vi "read_DAC.vi"() -> ()   [LabVIEW 2014]
uses:
  aardvark.dll
panel:
  out "Dup Aardvark Handle":i32
  out "DAC Val":u16 format="%.0x"
  in  "DAC_ADD":u16[](array[numeric]) format="%.0x"
  out "error out":errorcluster
  in  "error in (no error)":errorcluster
  in  "Address (0x50)":u16=80 max=1023 format="%.0x"
  in  "Aardvark Handle":i32 min=0
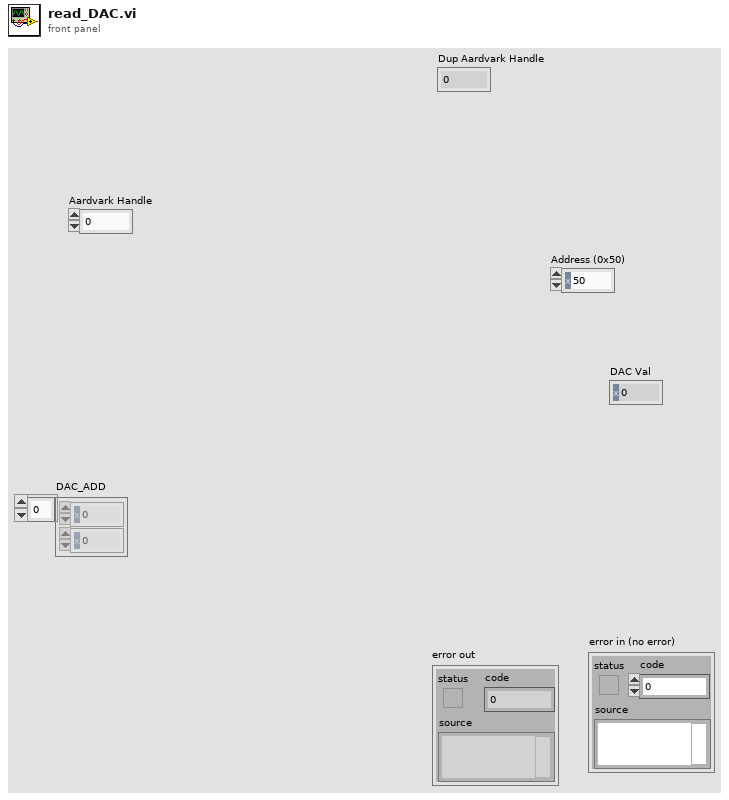
[diagram p1: front panel]
types:
  T1 = cluster{"Boolean array[0]":bool, "Boolean array[1]":bool, "Boolean array[2]":bool, "Boolean array[3]":bool, "Boolean array[4]":bool, "Boolean array[5]":bool, "Boolean array[6]":bool, "Boolean array[7]":bool}
  T2 = cluster{"Boolean array[0]":bool, "Boolean array[1]":bool, "Boolean array[2]":bool, "Boolean array[3]":bool, "Boolean array[4]":bool, "Boolean array[5]":bool, "Boolean array[6]":bool, "Boolean array[7]":bool, "Boolean array[0]":bool, "Boolean array[1]":bool, "Boolean array[2]":bool, "Boolean array[3]":bool}
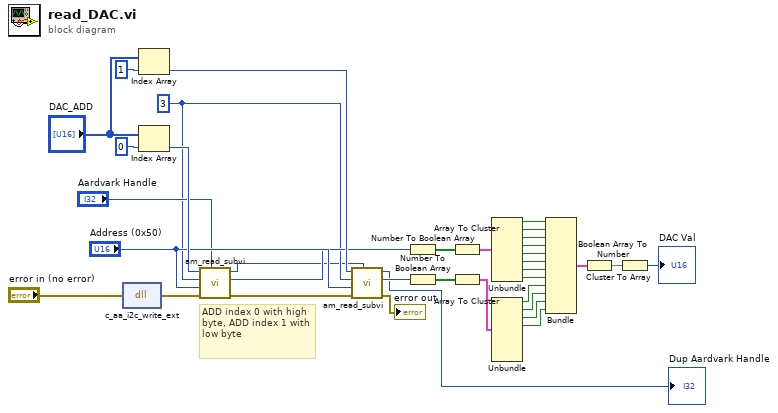
[diagram p0: block diagram]
diagram:
  w3 = u8 3
  # "ADD index 0 with high byte, ADD index 1 with low byte"
  n1 = dll-call lib="aardvark.dll" fn="c_aa_i2c_write_ext"(error in="error in (no error)") -> (error out=w30:errorcluster)  [unwired: 3 in, 1 out]
  n2 = Index Array(array="DAC_ADD", index=1) -> (element=w26:u16)
  n3 = Index Array(array="DAC_ADD", index=0) -> (element=w31:u16)
  n4 = call "am_read_subvi.vi"("Aardvark Handle in"="Aardvark Handle", "error in (no error)"=w30, "Address (0x50) in"="Address (0x50)", "Num Bytes to Fetch (64)"=w3, "Memory ADD"=w31) -> ("error out"=w29:errorcluster, "Data byte"=w4:u8, "Dup Aardvark Handle"=w2:i32)  [unwired: 4 in]
  n5 = call "am_read_subvi.vi"("Aardvark Handle in"=w2, "error in (no error)"=w29, "Address (0x50) in"="Address (0x50)", "Num Bytes to Fetch (64)"=w3, "Memory ADD"=w26) -> ("error out"=→"error out":errorcluster, "Data byte"=w5:u8, "Dup Aardvark Handle"=→"Dup Aardvark Handle":i32)  [unwired: 4 in]
  n6 = Number To Boolean Array(number=w4) -> (Boolean array=w23:bool[])
  n7 = Number To Boolean Array(number=w5) -> (Boolean array=w21:bool[])
  n8 = Array To Cluster(array=w23) -> (cluster=w24:T1)
  n9 = Array To Cluster(array=w21) -> (cluster=w22:T1)
  n10 = Unbundle(w24) -> ("Boolean array[0]"=w20:bool, "Boolean array[1]"=w19:bool, "Boolean array[2]"=w18:bool, "Boolean array[3]"=w17:bool, "Boolean array[4]"=w16:bool, "Boolean array[5]"=w15:bool, "Boolean array[6]"=w14:bool, "Boolean array[7]"=w13:bool)
  n11 = Unbundle(w22) -> ("Boolean array[0]"=w12:bool, "Boolean array[1]"=w11:bool, "Boolean array[2]"=w10:bool, "Boolean array[3]"=w9:bool)  [unwired: 4 out]
  n12 = Bundle("Boolean array[0]"=w20, "Boolean array[1]"=w19, "Boolean array[2]"=w18, "Boolean array[3]"=w17, "Boolean array[4]"=w16, "Boolean array[5]"=w15, "Boolean array[6]"=w14, "Boolean array[7]"=w13, "Boolean array[0]"=w12, "Boolean array[1]"=w11, "Boolean array[2]"=w10, "Boolean array[3]"=w9) -> (w8:T2)  [unwired: 1 in]
  n13 = Cluster To Array(cluster=w8) -> (array=w7:bool[])
  n14 = Boolean Array To Number(Boolean array=w7) -> (number=→"DAC Val":u32)
